vi "ABCDvec2SS.vi"(10 "Ndrift_p1":i16, 11 "ABCD_vec":dbl[](array[numeric])) -> (0 "error out":errorcluster, 2 "Gdrift":T1 {"Transport Delay" format="%.2f"; "D" format="%#.5g"; "C" format="%#.5g"; "B" format="%#.5g"; "A" format="%#.5g"; "properties"."Sampling Time" format="%#.6p"; "properties"."Output Delays" format="%.4f"; "properties"."Input Delays" format="%.4f"}, 3 "output array":dbl[][](array[numeric]))   [LabVIEW 2017]
uses:
  <vilib>/addons/Control Design/_Model Construction/Model Typedefs.llb/CD State Space Model (MIMO).ctl
  <vilib>/addons/Control Design/_Model Construction/Model Typedefs.llb/CD General Elements.ctl
  <vilib>/Analysis/Matrix/Numeric/Conversions/Array To Matrix - RA2.vi
  <vilib>/addons/Control Design/_Model Construction/Model Creation.llb/Model Creation SubVI/cd_Create State Space Model.vi
  <vilib>/addons/Control Design/_Model Construction/Model Information.llb/Model Information SubVIs/cd_Set Names To SS Model.vi
  <vilib>/Analysis/Matrix/NI_Matrix.lvlib
  <vilib>/addons/Control Design/_Model Construction/NI_LinSys_Model Creation.lvlib
  <vilib>/addons/Control Design/_Model Construction/NI_LinSys_Model Information.lvlib
  <vilib>/addons/Control Design/_Model Construction/NI_LinSys_Model Typedefs.lvlib
panel:
  in  "error in":errorcluster
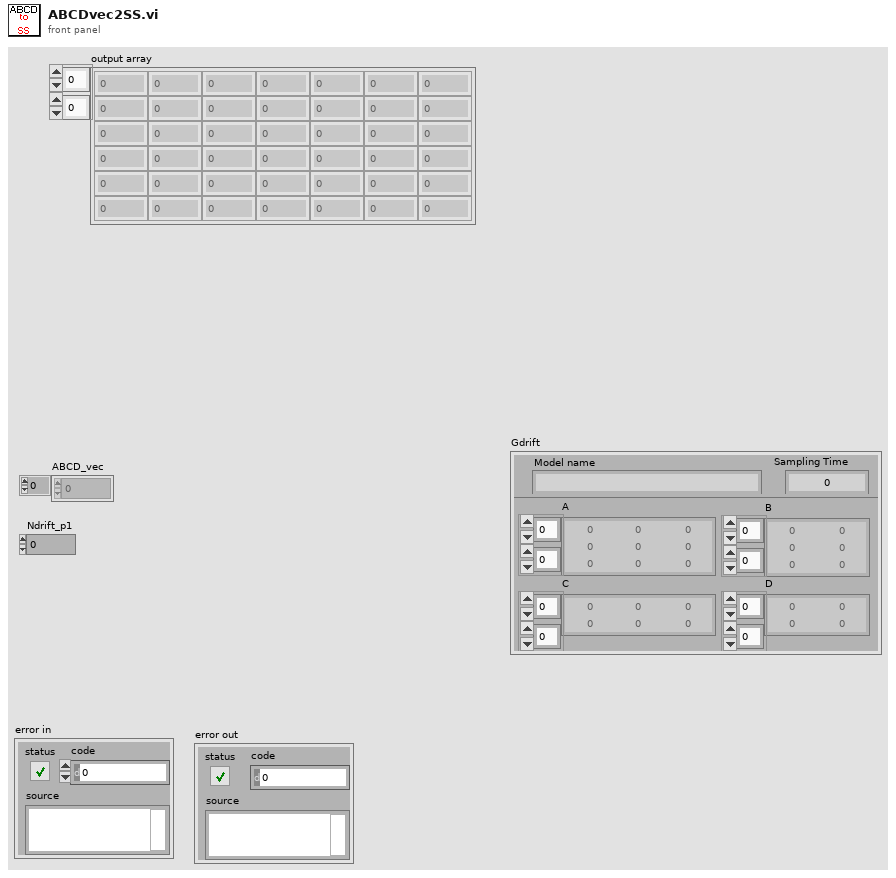
[diagram p1: front panel]
types:
  T1 = typedef "NI_LinSys_Model Typedefs.lvlib/CD State Space Model (MIMO).ctl" = cluster{"properties":T2, "A":dbl[][], "B":dbl[][], "C":dbl[][], "D":dbl[][], "StateNames":string[], "Transport Delay":dbl[][]}
  T2 = typedef "NI_LinSys_Model Typedefs.lvlib/CD General Elements.ctl" = cluster{"Model name":string, "Input names":string[], "Output names":string[], "Input Delays":dbl[], "Output Delays":dbl[], "Sampling Time":dbl, "Notes":string}
  T3 = typedef "NI_Matrix.lvlib/RealMatrix.ctl" = dbl[][]
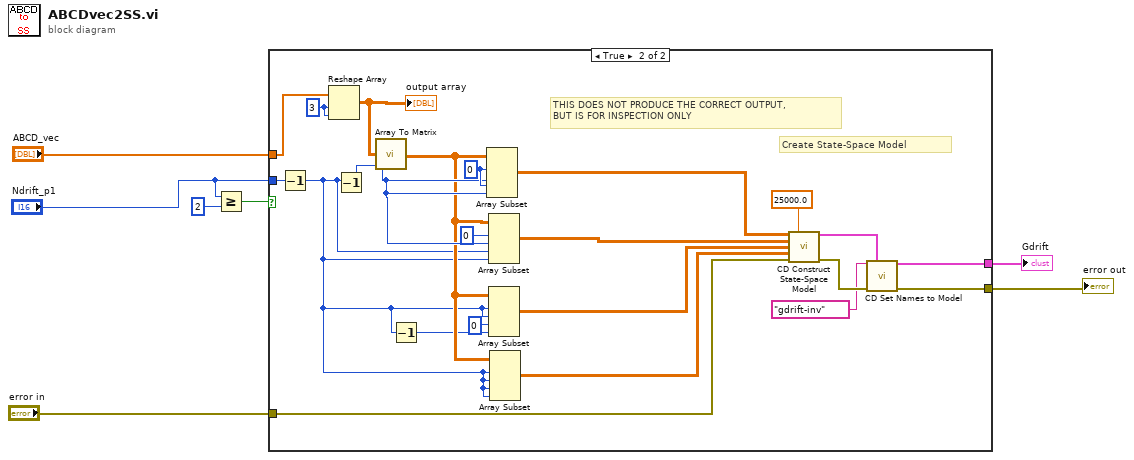
[diagram p0: block diagram]
diagram:
  n1 = Greater Or Equal?(x="Ndrift_p1", y=u8 2) -> (x >= y?=w1:bool)
  n2 = case shown="True" w1 {
    tunnel: [_ w15] -> w5
    tunnel: "Ndrift_p1" -> [_ w14]
    tunnel: "ABCD_vec" -> [_ w11]
    tunnel: [_ w13] -> w6
    tunnel: "error in" -> [_ w8]
    frame False {
    }
    frame True {
      w10 = 3 ("dimension size")
      w29 = 0 ("row 1")
      # "THIS DOES NOT PRODUCE THE CORRECT OUTPUT,\nBUT IS FOR INSPECTION ONLY"
      # "Create State-Space Model"
      n3 = Decrement(x=w14) -> (x-1=w20:i16)
      n4 = Reshape Array(w11, w10, w10) -> (w9:dbl[][])
      "output array" <- w9
      n5 = Decrement(x=w20) -> (x-1=w27:i16)
      n6 = call-poly <vilib>:"Array To Matrix.vi"("Real 2D Array"=w9) -> ("Real Matrix"=w24:T3)
      n7 = Decrement(x=w20) -> (x-1=w21:i16)
      n8 = Array Subset(array=w24, index (row)=w29, length (row)=w27, index (col)=w29, length (col)=w27) -> (w25:T3)
      n9 = Array Subset(array=w24, index (row)=0 ("row 1"), length (row)=w27, index (col)=w20, length (col)=w20) -> (w26:T3)
      n10 = Array Subset(array=w24, index (row)=w20, length (row)=w20, index (col)=0 ("row 1"), length (col)=w21) -> (w19:T3)
      n11 = Array Subset(array=w24, index (row)=w20, length (row)=w20, index (col)=w20, length (col)=w20) -> (w23:T3)
      n12 = call-poly <vilib>:"CD Construct State-Space Model.vi"("A"=w25, "Sampling Time (s)"=25000.0, "B"=w26, "C"=w19, "D"=w23, "error in (no error)"=w8) -> ("State-Space Model"=w16:T1, "error out"=w18:errorcluster)  [unwired: 8 in]
      n13 = call-poly <vilib>:"CD Set Names to Model.vi"("Model Name"="gdrift-inv", "State-Space Model In"=w16, "error in (no error)"=w18) -> ("Model Out"=w15:T1, "error out"=w13:errorcluster)  [unwired: 11 in]
    }
  }
  "Gdrift" <- w5
  "error out" <- w6
